vi "ProgramEEPROMwithTemp.vi"(8 "error in (no error)":errorcluster, 10 "reference":refnum<k7>, 11 "IN":T1={"step name 1"="", "updata 2"="1000", "limitdata 3"="", "load vi name 4"="", "parameter 5"=""}) -> (0 "error out":errorcluster, 2 "reference out":refnum<k7>, 3 "Cluster":T2)   [LabVIEW 2013]
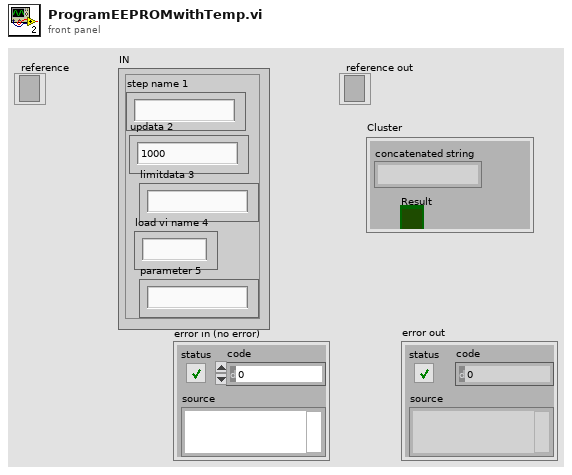
[diagram p1: front panel]
types:
  T1 = cluster{"step name 1":string, "updata 2":string, "limitdata 3":string, "load vi name 4":string, "parameter 5":string}
  T2 = cluster{"concatenated string":string, "Result":bool}
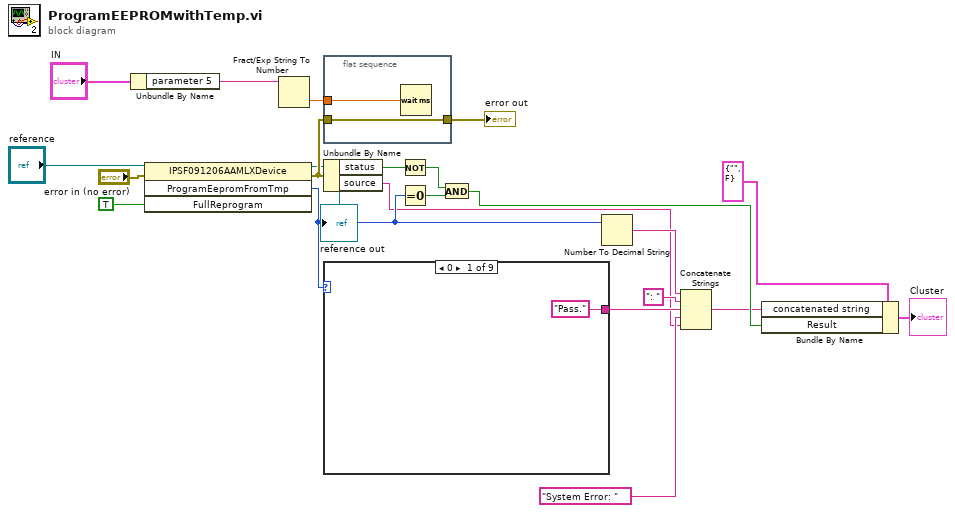
[diagram p0: block diagram]
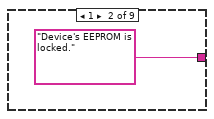
[diagram p2: hidden frame]
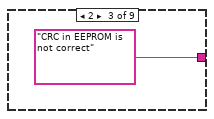
[diagram p3: hidden frame]
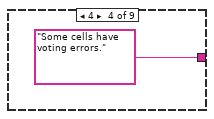
[diagram p4: hidden frame]
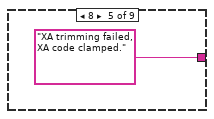
[diagram p5: hidden frame]
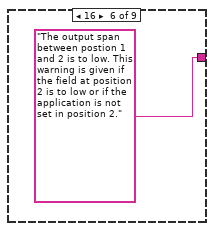
[diagram p6: hidden frame]
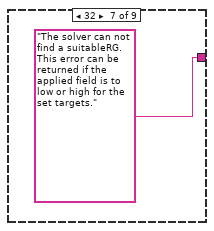
[diagram p7: hidden frame]
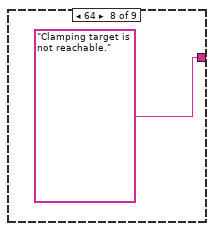
[diagram p8: hidden frame]
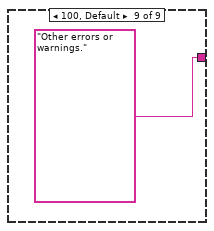
[diagram p9: hidden frame]
diagram:
  n1 = Unbundle By Name("IN") -> ("parameter 5"=w18:string)
  n2 = invoke class="IPSF091206AAMLXDevice" method="ProgramEepromFromTmp"(reference="reference", error in="error in (no error)", "FullReprogram"=TRUE) -> (reference out=→"reference out":refnum<k7>, error out=w4:errorcluster, "ProgramEepromFromTmp"=w11:i32)  [unwired: 1 in, 1 out]
  n3 = Fract/Exp String To Number(string=w18) -> (number=w19:dbl)  [unwired: 3 in, 1 out]
  n4 = flat-sequence {
    tunnel: w19 -> [w24]
    tunnel: w4 -> [w23]
    tunnel: [w23] -> w3
    frame #0 {
      n5 = Wait (ms)(milliseconds to wait=w24) -> ()  [unwired: 1 out]
    }
  }
  n6 = Unbundle By Name(w4) -> ("status"=w14:bool, "source"=w6:string)
  n7 = case shown="0" w11 {
    tunnel: ["Pass." "Device's EEPROM is locked." "CRC in EEPROM is not correct" "Some cells have voting errors." "XA trimming failed, XA code clamped." "The output span between postion 1 and 2 is to low. This warning is given if the field at position 2 is to low or if the application is not set in position 2." "The solver can not find a suitableRG. This error can be returned if the applied field is to low or high for the set targets." "Clamping target is not reachable." "Other errors or warnings."] -> w8
    frame 0 {
    }
    frame 1 {
    }
    frame 2 {
    }
    frame 4 {
    }
    frame 8 {
    }
    frame 16 {
    }
    frame 32 {
    }
    frame 64 {
    }
    frame 100, Default {
    }
  }
  n8 = Not(x=w14) -> (.not. x?=w13:bool)
  n9 = Equal To 0?(x=w11) -> (x = 0?=w15:bool)
  n10 = And(x=w13, y=w15) -> (x .and. y?=w12:bool)
  n11 = Number To Decimal String(number=w11) -> (decimal integer string=w10:string)  [unwired: 1 in]
  n12 = Concatenate Strings(w10, ": " ("string"), w8, "System Error: " ("string"), w6) -> (w5:string)
  n13 = Bundle By Name(cluster=T2 {"concatenated string"="", "Result"=FALSE} ("Cluster"), "concatenated string"=w5, "Result"=w12) -> (→"Cluster":T2)
  "error out" <- w3
